vi "Preview Direction StateQ.vi"(8 "error in (no error)":errorcluster, 9 "timeout in ms (-1)":i32, 11 "Cylinder in":refnum<class "Cylinder.lvclass">) -> (0 "error out":errorcluster, 1 "timed out?":bool, 2 "element":u16, 3 "Cylinder out":refnum<class "Cylinder.lvclass">, 4 "Valve StateQ":refnum<queue>)   [LabVIEW 2015, in "cRIO-Carbondioxide.lvlib" / "CO2-Actor.lvlib" / "Cylinder.lvclass"]
uses:
  Cylinder.lvclass
  Cylinder.lvclass/Cylinder.ctl
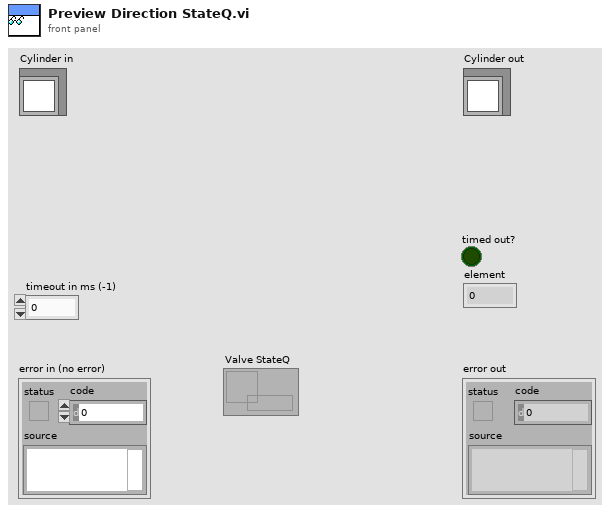
[diagram p1: front panel]
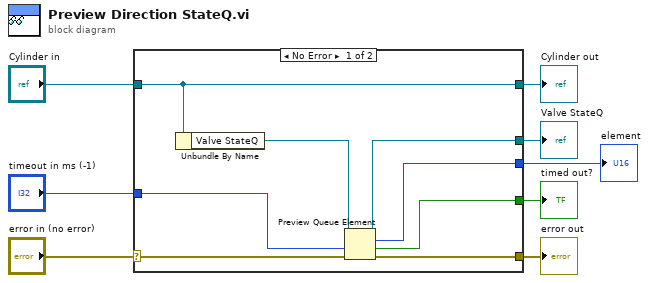
[diagram p0: block diagram]
diagram:
  n1 = case shown="No Error" "error in (no error)" {
    selector: "error in (no error)" -> [w15 w17]
    tunnel: [w14 w17] -> w7
    tunnel: [w16 w18] -> w5
    tunnel: "Cylinder in" -> [w16 w18]
    tunnel: [w11 _] -> w4
    tunnel: "timeout in ms (-1)" -> [w13 _]
    tunnel: [w10 _] -> w2
    tunnel: [w9 _] -> w1
    frame No Error {
      n2 = Unbundle By Name(w16) -> ("Valve StateQ"=w12:refnum<queue>)
      n3 = Preview Queue Element(queue=w12, timeout in ms (-1)=w13, error in (no error)=w15) -> (queue out=w11:refnum<queue>, element=w10:u16, timed out?=w9:bool, error out=w14:errorcluster)
    }
    frame Error {
    }
  }
  "error out" <- w7
  "Cylinder out" <- w5
  "Valve StateQ" <- w4
  "element" <- w2
  "timed out?" <- w1
